vi "Multichannel Recording0.9EP.vi"() -> ()   [LabVIEW 2014]
uses:
  Consumer Data_ Consumer Event Com.ctl
  Data Producer States.ctl
  Enum State Typedef.ctl
  <vilib>/_DAQmxBase/Internals/DAQmxBase Read (Analog 2D DBL NChan NSamp).vi
  <vilib>/_DAQmxBase/Internals/DAQmxBase Create Channel (AI-Voltage-Basic).vi
  <vilib>/_DAQmxBase/Internals/DAQmxBase Timing (Sample Clock).vi
panel:
  out "Recording Progress (% )":dbl(slide) scale=0.0..1.0
  in  "Display Size":T1(ring)
  out "Data Producer State":T2=enum."Default"
  out "Data Consumer State":T3=enum."Default"
  in  "Open Button":bool
  in  "Tab Control":T4(tab)
  in  "Amplifier Channel 0":T5 {"Amplifier Model" items=["Select a Model", "AM 1700", "BMA 200"]}
  out "Channel 0 Graph":waveform(dbl)(graph)
  in  "User Data Channel 0":T6
  in  "Use Channel 0":bool caption="In Use?"
  out "Channel 1 Graph":waveform(dbl)(graph)
  in  "User Data Channel 1":T6
  in  "Amplifier Channel 1":T5 {"Amplifier Model" items=["Select a Model", "AM 1700", "BMA 200"]}
  in  "Use Channel 1":bool caption="In Use?"
  out "Channel 2 Graph":waveform(dbl)(graph)
  in  "User Data Channel 2":T6
  in  "Amplifier Channel 2":T5 {"Amplifier Model" items=["Select a Model", "AM 1700", "BMA 200"]}
  in  "Use Channel 2":bool caption="In Use?"
  out "Channel 3 Graph":waveform(dbl)(graph)
  in  "User Data Channel 3":T6
  in  "Amplifier Channel 3":T5 {"Amplifier Model" items=["Select a Model", "AM 1700", "BMA 200"]}
  in  "Use Channel 3":bool caption="In Use?"
  out "Overview Graph":waveform(dbl)[](graph)
  in  "Stop Preview":bool
  in  "OK Button":bool
  in  "Clear Display":bool
  in  "Preview Button":bool
  in  "Recording Time (s)":dbl
  in  "Sample Rate":i64=1000
  in  "Stop Button":bool
  out "Start Time hr/min":string
  out "Date mm/dd/yy":string
  in  "Exit Button":bool
  in  "Record Button":bool
  # "MSU EFISH Lab Multi-Channel Electronic Pulse Recorder v0.9E (Beta 6)"
  # "Setup"
  # "Must set sample rate before you press start"
  # "Preview"
  # "Recording"
  # "Blue for On\nOrange for Off"
  # "DC"
  # "AC"
  # "Blue for AC and Orange for DC"
  # "Blue for On\nOrange for Off"
  # "DC"
  # "AC"
  # "Blue for AC and Orange for DC"
  # "Blue for On\nOrange for Off"
  # "DC"
  # "AC"
  # "Blue for AC and Orange for DC"
  # "Blue for On\nOrange for Off"
  # "DC"
  # "AC"
  # "Blue for AC and Orange for DC"
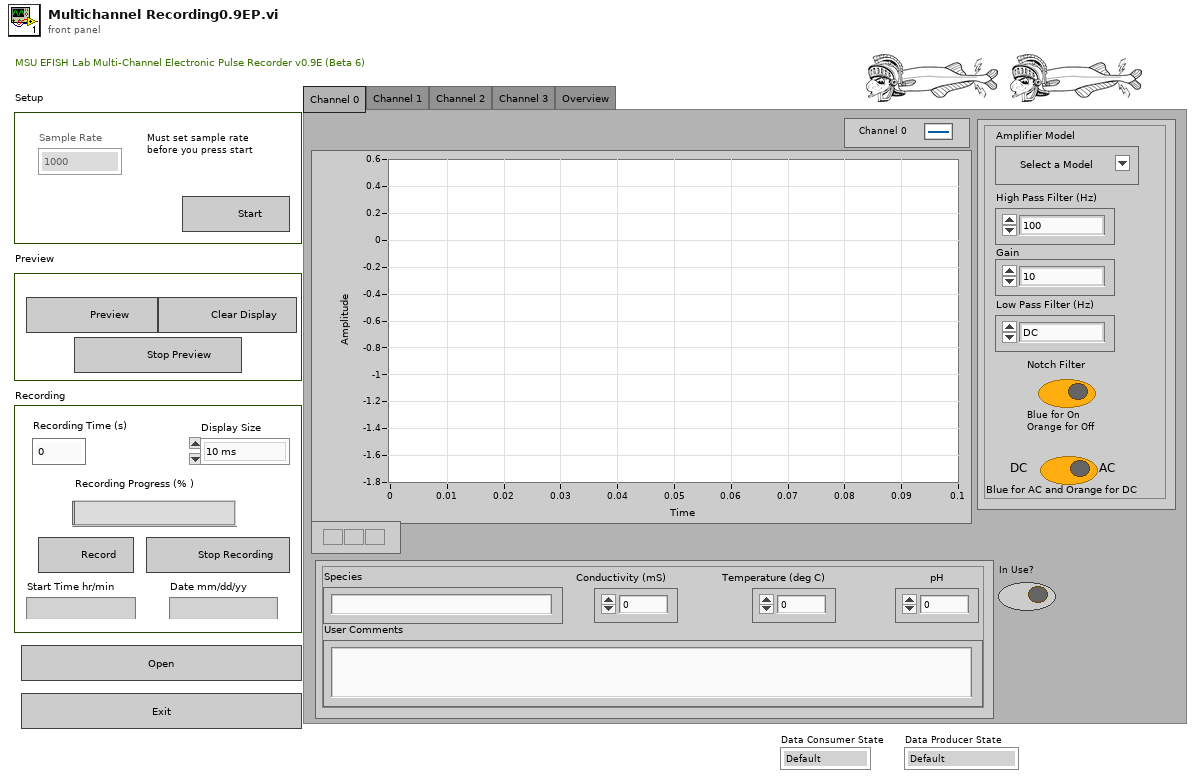
[diagram p1: front panel]
types:
  T1 = enum16{"10 ms", "100 ms", "1 Second", "10 sec", "30 sec"}
  T2 = typedef "Data Producer States.ctl" = enum16{"Read Data", "Set Sample Clock", "Default", "Exit", "Preview"}
  T3 = typedef "Consumer Data_ Consumer Event Com.ctl" = enum16{"Recording", "Create File", "Clear Memory", "Default", "End File", "Exit", "Set Sample Clock", "Preview"}
  T4 = enum32{"Channel 0", "Channel 1", "Channel 2", "Channel 3", "Overview"}
  T5 = cluster{"Low Pass Filter (Hz)":enum16{"DC", "0.1", "1", "3", "10", "30", "100", "300"}, "Gain ":enum16{"10", "20", "50", "100", "200", "500", "1000", "2k", "5k", "10k", "20k", "50k"}, "High Pass Filter (Hz)":enum16{"100", "500", "1000", "3000", "5000", "10,000", "20,000", "30,000", "50,000"}, "Notch Filter":bool, "Amplifier Model":u16, "AC/DC Switch":bool}
  T6 = cluster{"pH":dbl, "Conductivity (mS)":dbl, "Temperature (deg C)":dbl, "User Comments":string, "Species":string}
  T7 = enum8{"Enabled", "Disabled", "Disabled and Grayed Out"}
  T8 = cluster{"Overview Graph":refnum<vi>, "Channel 3 Graph":refnum<vi>, "Channel 2 Graph":refnum<vi>, "Channel 1 Graph":refnum<vi>, "Channel 0 Graph":refnum<vi>}
  T9 = typedef "Enum State Typedef.ctl" = enum16{"Default", "Open FIle", "Beginning State", "Set the Sample Clock", "Prepreview Handling", "Clear Display", "Preview Data", "Stop", "Exit", "Record", "Create File"}
  T10 = enum16{"Recording", "Create File", "Clear Memory", "Default"}
  T11 = cluster{"Refnum out":refnum<k34>, "Refnum out":refnum<k34>, "Refnum out":refnum<k34>, "Refnum out":refnum<k34>}
  T12 = cluster{"Use Channel 0":bool, "Use Channel 1":bool, "Use Channel 2":bool, "Use Channel 3":bool}
  T13 = cluster{"Waveform":waveform(dbl), "Waveform":waveform(dbl), "Waveform":waveform(dbl), "Waveform":waveform(dbl), waveform(dbl)[]}
  T14 = cluster{"tdms file out":refnum<k34>, "tdms file out":refnum<k34>, "tdms file out":refnum<k34>, "tdms file out":refnum<k34>}
  T15 = cluster{"User Data Channel 0":cluster{"pH":dbl, "Conductivity (mS)":dbl, "Temperature (deg C)":dbl, "User Comments":string, "Species":string}, "Amplifier Channel 0":cluster{"Low Pass Filter (Hz)":enum16{"DC", "0.1", "1", "3", "10", "30", "100", "300"}, "Gain ":enum16{"10", "20", "50", "100", "200", "500", "1000", "2k", "5k", "10k", "20k", "50k"}, "High Pass Filter (Hz)":enum16{"100", "500", "1000", "3000", "5000", "10,000", "20,000", "30,000", "50,000"}, "Notch Filter":bool, "Amplifier Model":u16, "AC/DC Switch":bool}, "User Data Channel 1":cluster{"pH":dbl, "Conductivity (mS)":dbl, "Temperature (deg C)":dbl, "User Comments":string, "Species":string}, "Amplifier Channel 1":cluster{"Low Pass Filter (Hz)":enum16{"DC", "0.1", "1", "3", "10", "30", "100", "300"}, "Gain ":enum16{"10", "20", "50", "100", "200", "500", "1000", "2k", "5k", "10k", "20k", "50k"}, "High Pass Filter (Hz)":enum16{"100", "500", "1000", "3000", "5000", "10,000", "20,000", "30,000", "50,000"}, "Notch Filter":bool, "Amplifier Model":u16, "AC/DC Switch":bool}, "User Data Channel 2":cluster{"pH":dbl, "Conductivity (mS)":dbl, "Temperature (deg C)":dbl, "User Comments":string, "Species":string}, "Amplifier Channel 2":cluster{"Low Pass Filter (Hz)":enum16{"DC", "0.1", "1", "3", "10", "30", "100", "300"}, "Gain ":enum16{"10", "20", "50", "100", "200", "500", "1000", "2k", "5k", "10k", "20k", "50k"}, "High Pass Filter (Hz)":enum16{"100", "500", "1000", "3000", "5000", "10,000", "20,000", "30,000", "50,000"}, "Notch Filter":bool, "Amplifier Model":u16, "AC/DC Switch":bool}, "User Data Channel 3":cluster{"pH":dbl, "Conductivity (mS)":dbl, "Temperature (deg C)":dbl, "User Comments":string, "Species":string}, "Amplifier Channel 3":cluster{"Low Pass Filter (Hz)":enum16{"DC", "0.1", "1", "3", "10", "30", "100", "300"}, "Gain ":enum16{"10", "20", "50", "100", "200", "500", "1000", "2k", "5k", "10k", "20k", "50k"}, "High Pass Filter (Hz)":enum16{"100", "500", "1000", "3000", "5000", "10,000", "20,000", "30,000", "50,000"}, "Notch Filter":bool, "Amplifier Model":u16, "AC/DC Switch":bool}}
  T16 = enum16{"Read Data", "Set Sample Clock", "Default", "Exit"}
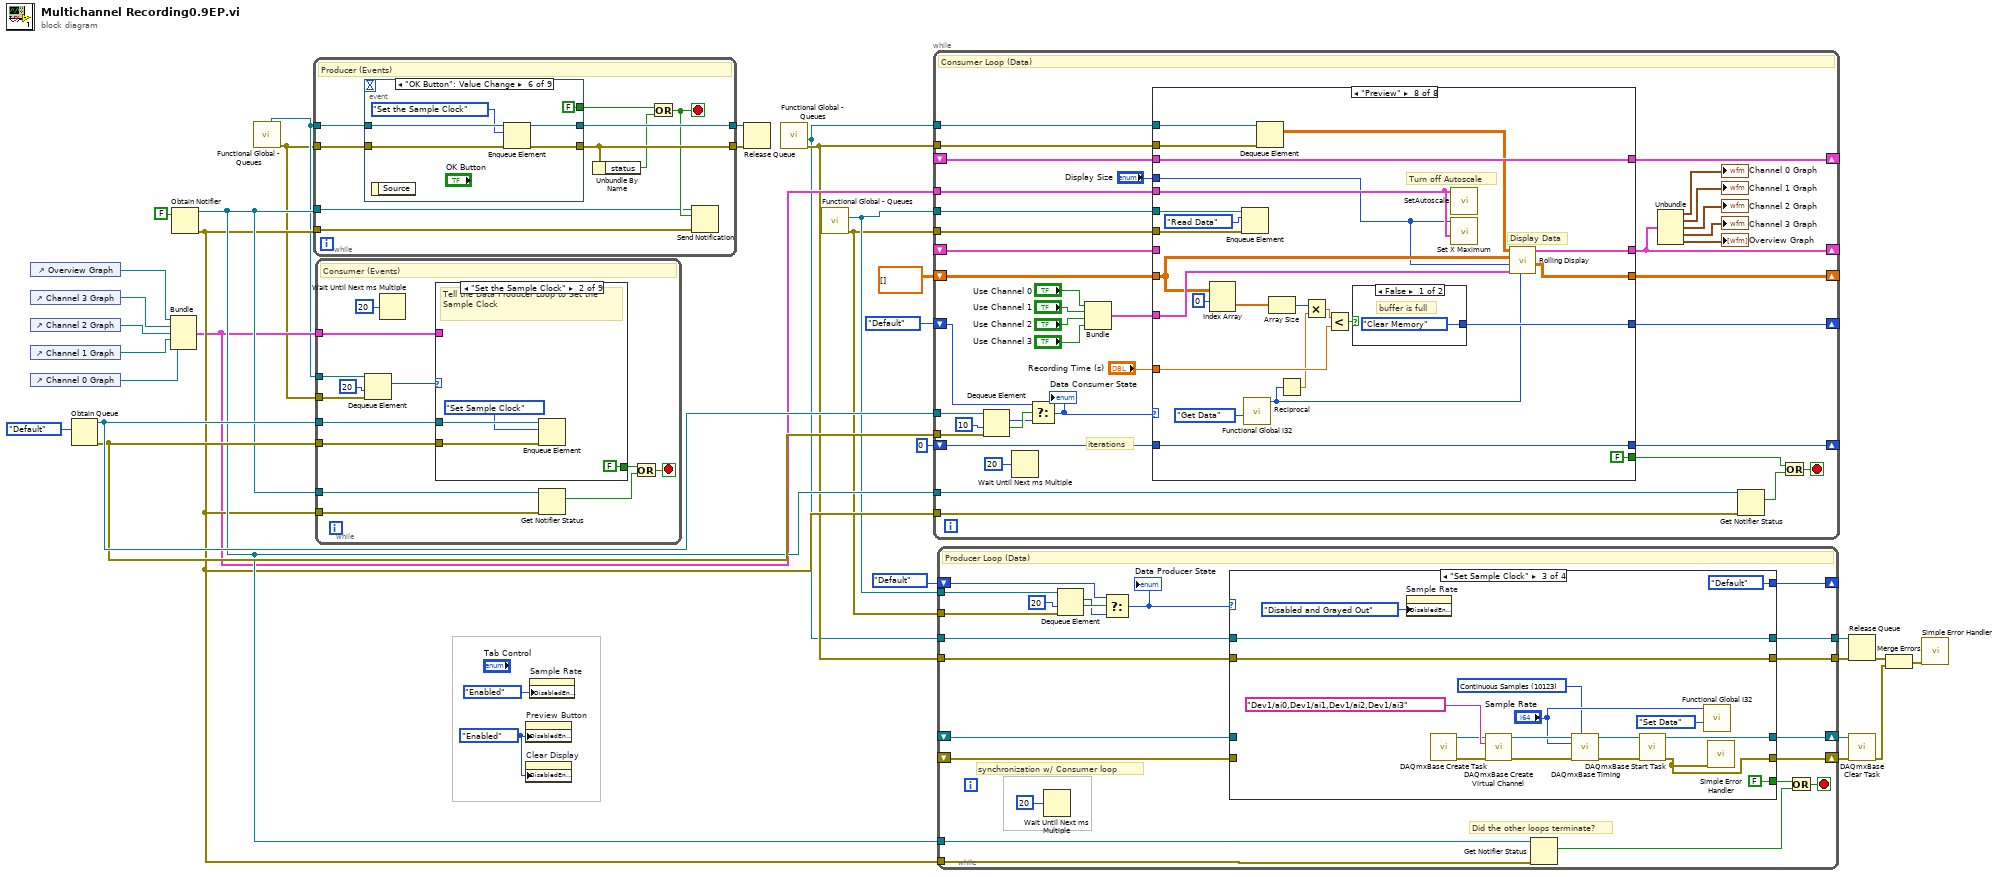
[diagram p0: block diagram]
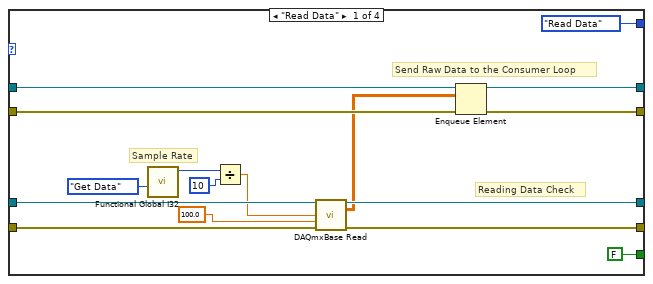
[diagram p2: hidden frame]
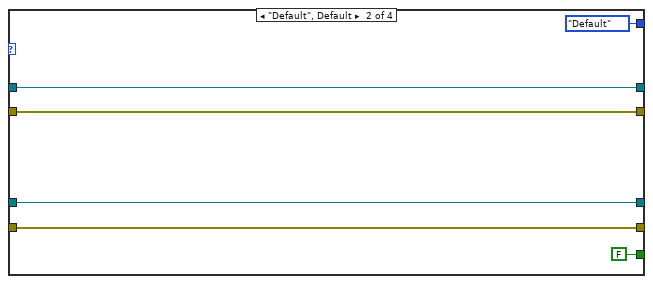
[diagram p3: hidden frame]
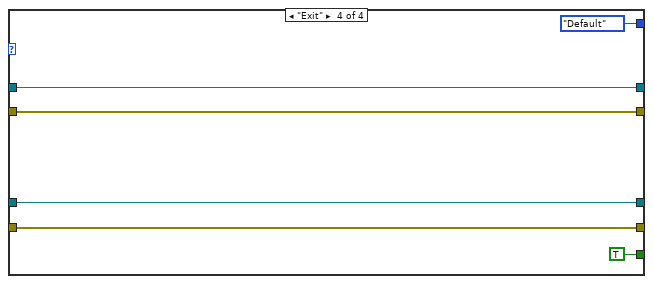
[diagram p4: hidden frame]
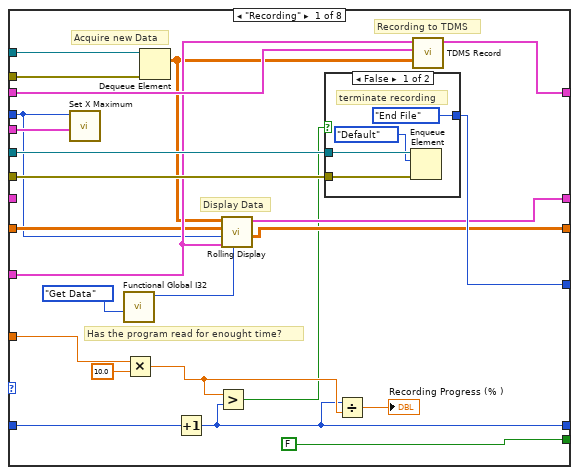
[diagram p5: hidden frame]
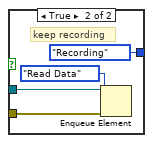
[diagram p6: hidden frame]
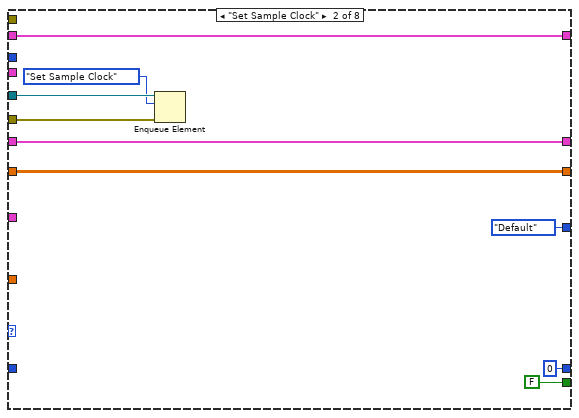
[diagram p7: hidden frame]
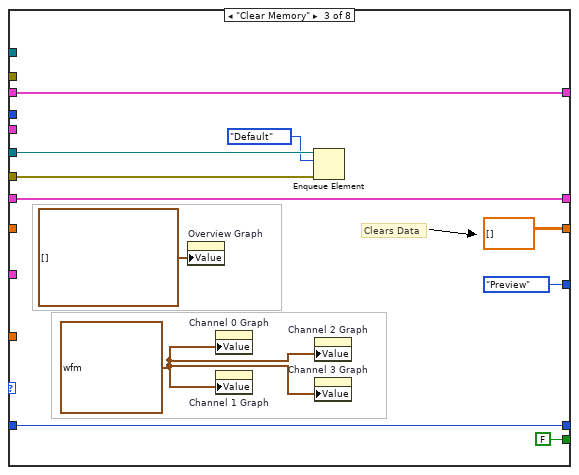
[diagram p8: hidden frame]
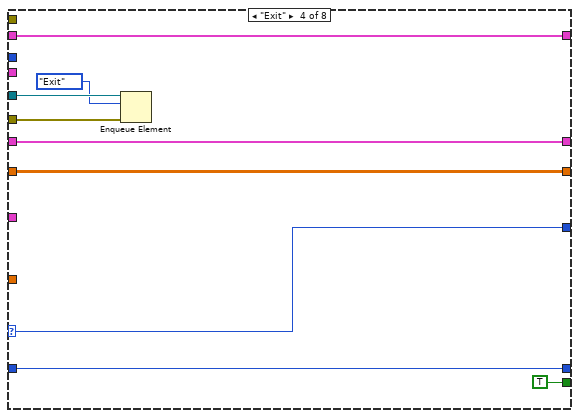
[diagram p9: hidden frame]
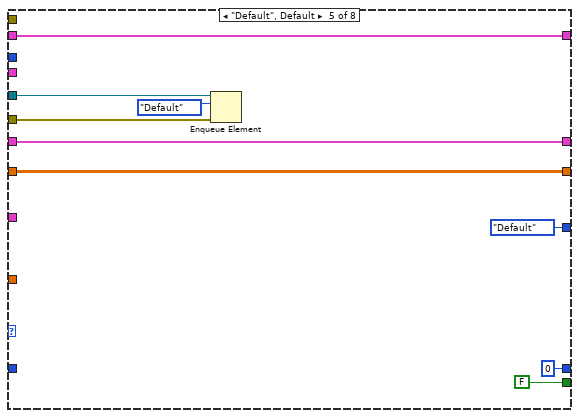
[diagram p10: hidden frame]
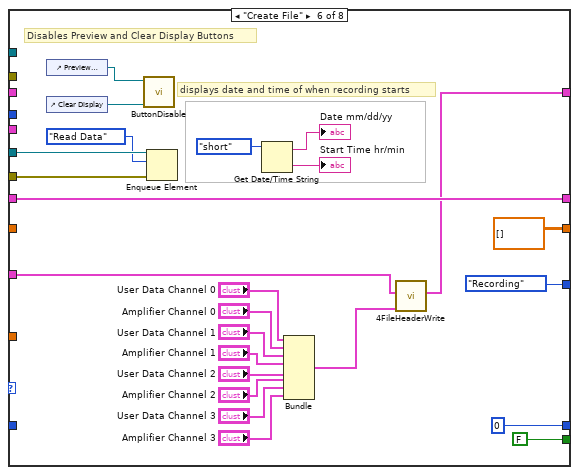
[diagram p11: hidden frame]
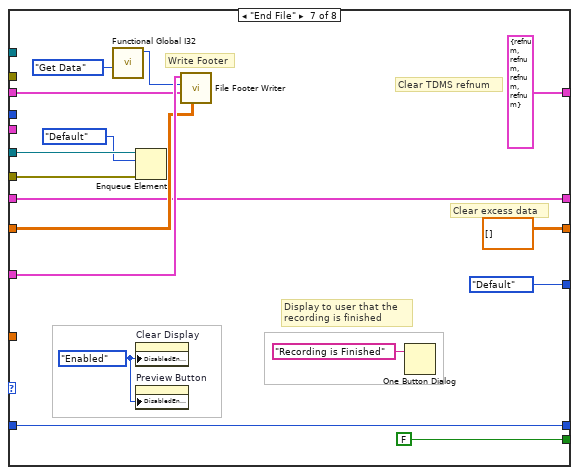
[diagram p12: hidden frame]
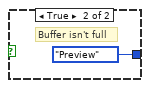
[diagram p13: hidden frame]
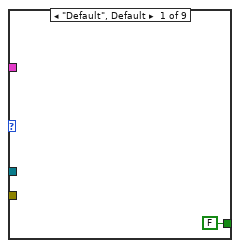
[diagram p14: hidden frame]
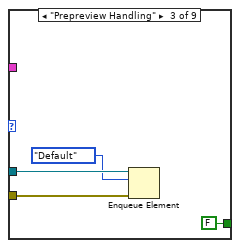
[diagram p15: hidden frame]
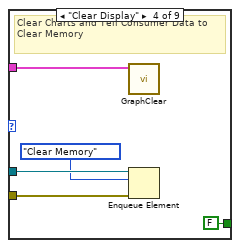
[diagram p16: hidden frame]
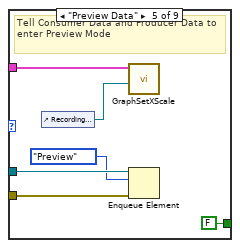
[diagram p17: hidden frame]
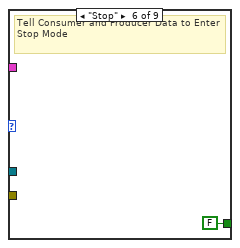
[diagram p18: hidden frame]
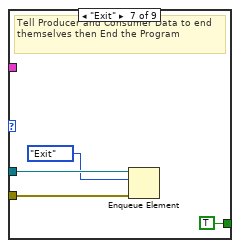
[diagram p19: hidden frame]
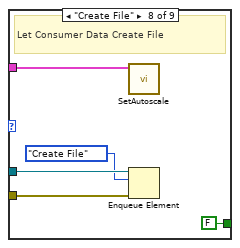
[diagram p20: hidden frame]
diagram:
  w13 = T7."Enabled" ("Disabled")
  n1 = control-ref of="Overview Graph"() -> (w12:refnum<vi>)
  n2 = control-ref of="Channel 3 Graph"() -> (w11:refnum<vi>)
  n3 = control-ref of="Channel 2 Graph"() -> (w10:refnum<vi>)
  n4 = control-ref of="Channel 1 Graph"() -> (w9:refnum<vi>)
  n5 = control-ref of="Channel 0 Graph"() -> (w8:refnum<vi>)
  n6 = Obtain Queue(element data type=Consumer_Data__Consumer_Event_Com."Default") -> (queue out=w29:refnum<queue>, error out=w28:errorcluster)  [unwired: 4 in, 1 out]
  n7 = Bundle("Overview Graph"=w12, "Channel 3 Graph"=w11, "Channel 2 Graph"=w10, "Channel 1 Graph"=w9, "Channel 0 Graph"=w8) -> (w7:T8)  [unwired: 1 in]
  n8 = Obtain Notifier(notification data type=FALSE) -> (notifier out=w15:refnum<notifier>, error out=w14:errorcluster)  [unwired: 3 in, 1 out]
  n9 = call "Functional Global - Queues.vi"() -> ("Error Out"=w1:errorcluster, "Producer Consumer Events Q"=w2:refnum<queue>)  [unwired: 7 in, 3 out]
  n10 = while {
    tunnel: w2 -> [w42]
    tunnel: w1 -> [w41]
    tunnel: [w40] -> w33
    tunnel: [w39] -> w32
    tunnel: w15 -> [w35]
    tunnel: w14 -> [w34]
    stop <- w36 stop-if-true
    # "Producer (Events)"
    n11 = event shown="[5] \"OK Button\": Value Change" {
      selector: _ -> [_ _ _ _ _ _ _ _ _]
      dyn-events: _ -> [_ _ _ _ _ _ _ _ _]
      timeout: _ -> [_ _ _ _ _ _ _ _ _]
      tunnel: [FALSE ("Exit Button") "Exit Button" FALSE ("Exit Button") FALSE ("Exit Button") FALSE ("Exit Button") FALSE ("Exit Button") FALSE ("Exit Button") FALSE ("Exit Button") FALSE ("Exit Button")] -> w38
      tunnel: w42 -> [w44 w50 w57 w63 w69 w75 w81 w87 w93]
      tunnel: w41 -> [w43 w49 w56 w62 w68 w74 w80 w86 w92]
      tunnel: [w44 w47 w53 w59 w65 w71 w77 w83 w89] -> w40
      tunnel: [w43 w46 w52 w58 w64 w70 w76 w82 w88] -> w39
      event Timeout {
        n12 = event-data() -> ()  [unwired: 1 in, 1 out]
      }
      event "Exit Button": Value Change {
        n13 = event-data() -> ()  [unwired: 1 in, 1 out]
        n14 = Enqueue Element(queue=w50, element=Enum_State_Typedef."Exit", error in (no error)=w49) -> (queue out=w47:refnum<queue>, error out=w46:errorcluster)  [unwired: 1 in, 1 out]
      }
      event "Preview Button": Value Change {
        n15 = event-data() -> ()  [unwired: 1 in, 1 out]
        n16 = Enqueue Element(queue=w57, element=Enum_State_Typedef."Preview Data", error in (no error)=w56) -> (queue out=w53:refnum<queue>, error out=w52:errorcluster)  [unwired: 1 in, 1 out]
      }
      event "Stop Preview": Value Change {
        n17 = event-data() -> ()  [unwired: 1 in, 1 out]
        n18 = Enqueue Element(queue=w63, element=Enum_State_Typedef."Prepreview Handling", error in (no error)=w62) -> (queue out=w59:refnum<queue>, error out=w58:errorcluster)  [unwired: 1 in, 1 out]
      }
      event "Open Button": Value Change {
        n19 = event-data() -> ()  [unwired: 1 in, 1 out]
        n20 = Enqueue Element(queue=w69, element=Enum_State_Typedef."Open FIle", error in (no error)=w68) -> (queue out=w65:refnum<queue>, error out=w64:errorcluster)  [unwired: 1 in, 1 out]
      }
      event "OK Button": Value Change {
        n21 = event-data() -> ()  [unwired: 1 in, 1 out]
        n22 = Enqueue Element(queue=w75, element=Enum_State_Typedef."Set the Sample Clock", error in (no error)=w74) -> (queue out=w71:refnum<queue>, error out=w70:errorcluster)  [unwired: 1 in, 1 out]
      }
      event "Stop Button": Value Change {
        n23 = event-data() -> ()  [unwired: 1 in, 1 out]
        n24 = Enqueue Element(queue=w81, element=Enum_State_Typedef."Stop", error in (no error)=w80) -> (queue out=w77:refnum<queue>, error out=w76:errorcluster)  [unwired: 1 in, 1 out]
      }
      event "Record Button": Value Change {
        n25 = event-data() -> ()  [unwired: 1 in, 1 out]
        n26 = Enqueue Element(queue=w87, element=Enum_State_Typedef."Create File", error in (no error)=w86) -> (queue out=w83:refnum<queue>, error out=w82:errorcluster)  [unwired: 1 in, 1 out]
      }
      event "Clear Display": Value Change {
        n27 = event-data() -> ()  [unwired: 1 in, 1 out]
        n28 = Enqueue Element(queue=w93, element=Enum_State_Typedef."Clear Display", error in (no error)=w92) -> (queue out=w89:refnum<queue>, error out=w88:errorcluster)  [unwired: 1 in, 1 out]
      }
    }
    n29 = Unbundle By Name(w39) -> ("status"=w37:bool)
    n30 = Or(x=w38, y=w37) -> (x .or. y?=w36:bool)
    n31 = Send Notification(notification=w36, notifier=w35, error in (no error)=w34) -> ()  [unwired: 2 out]
  }
  n32 = while {
    tunnel: w2 -> [w106]
    tunnel: w1 -> [w105]
    tunnel: w29 -> [w104]
    tunnel: w28 -> [w103]
    tunnel: w15 -> [w98]
    tunnel: w14 -> [w97]
    tunnel: w7 -> [w94]
    stop <- w96 stop-if-true
    # "Consumer (Events)"
    n33 = Dequeue Element(queue=w106, timeout in ms (-1)=20, error in (no error)=w105) -> (element=w101:T9)  [unwired: 3 out]
    n34 = Wait Until Next ms Multiple(millisecond multiple=u32 20) -> ()  [unwired: 1 out]
    n35 = case shown="\"Set the Sample Clock\"" w101 {
      tunnel: w104 -> [_ w110 w114 w119 w125 _ w131 w135 _]
      tunnel: w103 -> [_ w109 w113 w118 w124 _ w130 w134 _]
      tunnel: [FALSE FALSE FALSE FALSE FALSE FALSE TRUE FALSE FALSE] -> w102
      tunnel: w94 -> [_ _ _ w116 w121 _ _ w132 _]
      frame "Default", Default {
      }
      frame "Set the Sample Clock" {
        # "Tell the Data Producer Loop to Set the Sample Clock"
        n36 = Enqueue Element(queue=w110, element=Consumer_Data__Consumer_Event_Com."Set Sample Clock", error in (no error)=w109) -> ()  [unwired: 1 in, 3 out]
      }
      frame "Prepreview Handling" {
        n37 = Enqueue Element(queue=w114, element=Consumer_Data__Consumer_Event_Com."Default", error in (no error)=w113) -> ()  [unwired: 1 in, 3 out]
      }
      frame "Clear Display" {
        # "Clear Charts and Tell Consumer Data to Clear Memory"
        n38 = call "GraphClear.vi"("Graph Reference Cluster"=w116) -> ()  [unwired: 11 in]
        n39 = Enqueue Element(queue=w119, element=Consumer_Data__Consumer_Event_Com."Clear Memory", error in (no error)=w118) -> ()  [unwired: 1 in, 3 out]
      }
      frame "Preview Data" {
        # "Tell Consumer Data and Producer Data to enter Preview Mode"
        n40 = control-ref of="Recording Time (s)"() -> (w122:refnum<vi>)
        n41 = call "GraphSetXScale.vi"("Graph Reference Cluster"=w121, "Recording Time Reference"=w122) -> ()  [unwired: 9 in]
        n42 = Enqueue Element(queue=w125, element=Consumer_Data__Consumer_Event_Com."Preview", error in (no error)=w124) -> ()  [unwired: 1 in, 3 out]
      }
      frame "Stop" {
        # "Tell Consumer and Producer Data to Enter Stop Mode"
      }
      frame "Exit" {
        # "Tell Producer and Consumer Data to end themselves then End the Program"
        n43 = Enqueue Element(queue=w131, element=Consumer_Data__Consumer_Event_Com."Exit", error in (no error)=w130) -> ()  [unwired: 1 in, 3 out]
      }
      frame "Create File" {
        # "Let Consumer Data Create File"
        n44 = call "SetAutoscale.vi"("Graph Reference Cluster"=w132) -> ()  [unwired: 11 in]
        n45 = Enqueue Element(queue=w135, element=Consumer_Data__Consumer_Event_Com."Create File", error in (no error)=w134) -> ()  [unwired: 1 in, 3 out]
      }
      frame "Open FIle" {
        # "Tell the Data Consumer to Create the File"
        n46 = call "File Dialog"() -> ("selected path"=w137:path)  [unwired: 12 in, 3 out]
        n47 = call <vilib>:"TDMS - File Viewer.vi"("file path"=w137) -> ()  [unwired: 5 in, 2 out]
      }
    }
    n48 = Get Notifier Status(notifier=w98, error in (no error)=w97) -> (current notification=w95:bool)  [unwired: 4 out]
    n49 = Or(x=w102, y=w95) -> (x .or. y?=w96:bool)
  }
  n50 = property on="Preview Button" class="Bool (strict)"("DisabledEnum"=w13) -> ()  [unwired: 2 in, 2 out]
  n51 = property on="Clear Display" class="Bool"("DisabledEnum"=w13) -> ()  [unwired: 2 in, 2 out]
  n52 = property on="Sample Rate" class="DigNum (strict)"("DisabledEnum"=T7."Enabled" ("Disabled")) -> ()  [unwired: 2 in, 2 out]
  n53 = Release Queue(queue=w33, error in (no error)=w32) -> ()  [unwired: 1 in, 3 out]
  n54 = call "Functional Global - Queues.vi"() -> ("Error Out"=w6:errorcluster, "Data Q"=w5:refnum<queue>)  [unwired: 7 in, 3 out]
  n55 = call "Functional Global - Queues.vi"() -> ("Error Out"=w3:errorcluster, "Data Producer Control Q"=w4:refnum<queue>)  [unwired: 7 in, 3 out]
  n56 = while {
    tunnel: w5 -> [w170]
    tunnel: w6 -> [w169]
    tunnel: w29 -> [w177]
    tunnel: w28 -> [w176]
    shift-right: [w171] -> _
    shift-left: Consumer_Data__Consumer_Event_Com."Default" -> [w172]
    shift-right: [w165] -> _
    shift-left: dbl[][] [] -> [w168]
    shift-right: [w164] -> _
    shift-left: _ -> [w163]
    tunnel: w4 -> [w161]
    tunnel: w3 -> [w160]
    shift-right: [w156] -> _
    shift-left: 0 -> [w158]
    tunnel: w15 -> [w150]
    tunnel: w14 -> [w149]
    shift-right: [w142] -> _
    shift-left: _ -> [w141]
    tunnel: w7 -> [w139]
    stop <- w152 stop-if-true
    # "iterations"
    # "Consumer Loop (Data)"
    n57 = Dequeue Element(queue=w177, timeout in ms (-1)=10, error in (no error)=w176) -> (element=w174:T3, timed out?=w175:bool)  [unwired: 2 out]
    n58 = Wait Until Next ms Multiple(millisecond multiple=u32 20) -> ()  [unwired: 1 out]
    n59 = Select(t=w172, s=w175, f=w174) -> (s? t:f=w173:T3)
    "Data Consumer State" <- w173
    n60 = Bundle("Use Channel 0"="Use Channel 0", "Use Channel 1"="Use Channel 1", "Use Channel 2"="Use Channel 2", "Use Channel 3"="Use Channel 3") -> (w166:T12)  [unwired: 1 in]
    n61 = case shown="\"Preview\"" w173 {
      selector: w173 -> [_ _ _ w236 _ _ _ _]
      tunnel: [w194 Consumer_Data__Consumer_Event_Com."Default" Consumer_Data__Consumer_Event_Com."Preview" w236 T10."Default" Consumer_Data__Consumer_Event_Com."Recording" Consumer_Data__Consumer_Event_Com."Default" w306] -> w171
      tunnel: w170 -> [w200 _ _ _ _ _ _ w312]
      tunnel: w169 -> [w199 _ _ _ _ _ _ w311]
      tunnel: [FALSE FALSE FALSE TRUE FALSE FALSE FALSE FALSE] -> w151
      tunnel: w168 -> [w180 w215 _ w237 w245 _ w285 w293]
      tunnel: w166 -> [w189 _ _ _ _ w250 w287 w298]
      tunnel: [w187 w215 dbl[][] [] ("Output Decimated Data") w237 w245 dbl[][] [] ("Output Decimated Data") dbl[][] [] ("Output Data") w296] -> w165
      tunnel: [w198 w214 w226 w235 w244 w252 T11 {"Refnum out"=refnum, "Refnum out"=refnum, "Refnum out"=refnum, "Refnum out"=refnum} ("Output TDMS File Cluster") w299] -> w164
      tunnel: w163 -> [w191 w214 w226 w235 w244 _ w286 w299]
      tunnel: w161 -> [w193 w218 w225 w234 w242 w265 w280 w304]
      tunnel: w160 -> [w192 w217 w224 w233 w241 w264 w279 w303]
      tunnel: w158 -> [w197 _ w222 w231 _ _ w277 w301]
      tunnel: "Recording Time (s)" -> [w196 _ _ _ _ _ _ w294]
      tunnel: [w183 0 w222 w231 0 0 w277 w301] -> w156
      tunnel: [w188 w210 w221 w230 w239 w261 w275 w297] -> w142
      tunnel: w141 -> [_ w210 w221 w230 w239 w261 w275 _]
      tunnel: "Display Size" -> [w179 _ _ _ _ _ _ w290]
      tunnel: w139 -> [w185 _ _ _ _ _ _ w295]
      frame "Recording" {
        # "Acquire new Data"
        # "Has the program read for enought time?"
        # "Display Data"
        # "Recording to TDMS"
        n62 = call "Set X Maximum.vi"("Graph Reference Cluster"=w185, "Display Size"=w179) -> ()  [unwired: 10 in]
        n63 = call "Functional Global I32.vi"("Enum"=enum16{"Set Data", "Get Data"}."Get Data") -> ("Integer"=w178:i32)  [unwired: 10 in]
        n64 = Multiply(x=w196, y=10.0) -> (x*y=w184:dbl)
        n65 = Dequeue Element(queue=w200, error in (no error)=w199) -> (element=w181:dbl[][])  [unwired: 1 in, 3 out]
        n66 = Increment(x=w197) -> (x+1=w183:i32)
        n67 = Greater?(x=w184, y=w183) -> (0:w182:bool)
        n68 = call "Rolling Display.vi"("Sample Rate"=w178, "Channels in Use"=w189, "Display Size"=w179, "Old Data"=w180, "Input Data"=w181) -> ("Output Array Values"=w187:dbl[][], "Output Waveform Cluster"=w188:T13)  [unwired: 5 in]
        n69 = case shown="False" w182 {
          tunnel: [Consumer_Data__Consumer_Event_Com."End File" Consumer_Data__Consumer_Event_Com."Recording"] -> w194
          tunnel: w193 -> [w204 w208]
          tunnel: w192 -> [w203 w207]
          frame False {
            # "terminate recording"
            n70 = Enqueue Element(queue=w204, element=Data_Producer_States."Default", error in (no error)=w203) -> ()  [unwired: 1 in, 3 out]
          }
          frame True {
            # "keep recording"
            n71 = Enqueue Element(queue=w208, element=Data_Producer_States."Read Data", error in (no error)=w207) -> ()  [unwired: 1 in, 3 out]
          }
        }
        n72 = Divide(x=w183, y=w184) -> (x/y=→"Recording Progress (% )":dbl)
        n73 = call "TDMS Record.vi"("Data"=w181, "Input TDMS File Cluster"=w191, "In Use Cluster"=w189) -> ("Output TDMS File Cluster"=w198:T14)  [unwired: 8 in]
      }
      frame "Set Sample Clock" {
        n74 = Enqueue Element(queue=w218, element=Data_Producer_States."Set Sample Clock", error in (no error)=w217) -> ()  [unwired: 1 in, 3 out]
      }
      frame "Clear Memory" {
        w220 = waveform(dbl) {"t0"=timestamp(0 s since 1904-01-01), "dt"=1.0, "Y"=[]} ("Channel 0 Graph")
        # "Clears Data"
        n75 = property on="Overview Graph" class="WFGraph (strict)"("Value"=waveform(dbl)[] [] ("Overview Graph")) -> ()  [unwired: 2 in, 2 out]
        n76 = property on="Channel 0 Graph" class="WFGraph (strict)"("Value"=w220) -> ()  [unwired: 2 in, 2 out]
        n77 = property on="Channel 1 Graph" class="WFGraph (strict)"("Value"=w220) -> ()  [unwired: 2 in, 2 out]
        n78 = Enqueue Element(queue=w225, element=Data_Producer_States."Default", error in (no error)=w224) -> ()  [unwired: 1 in, 3 out]
        n79 = property on="Channel 2 Graph" class="WFGraph (strict)"("Value"=w220) -> ()  [unwired: 2 in, 2 out]
        n80 = property on="Channel 3 Graph" class="WFGraph (strict)"("Value"=w220) -> ()  [unwired: 2 in, 2 out]
      }
      frame "Exit" {
        n81 = Enqueue Element(queue=w234, element=Data_Producer_States."Exit", error in (no error)=w233) -> ()  [unwired: 1 in, 3 out]
      }
      frame "Default", Default {
        n82 = Enqueue Element(queue=w242, element=Data_Producer_States."Default", error in (no error)=w241) -> ()  [unwired: 1 in, 3 out]
      }
      frame "Create File" {
        # "displays date and time of when recording starts"
        # "Disables Preview and Clear Display Buttons"
        n83 = control-ref of="Preview Button"() -> (w248:refnum<vi>)
        n84 = control-ref of="Clear Display"() -> (w249:refnum<vi>)
        n85 = call "ButtonDisable.vi"("Clear Display Button Reference"=w249, "Preview Button Reference"=w248) -> ()  [unwired: 10 in]
        n86 = Enqueue Element(queue=w265, element=Data_Producer_States."Read Data", error in (no error)=w264) -> ()  [unwired: 1 in, 3 out]
        n87 = Get Date/Time String(date format (0)=enum16{"short", "long", "abbreviated"}."short") -> (date string=→"Date mm/dd/yy":string, time string=→"Start Time hr/min":string)  [unwired: 2 in]
        n88 = Bundle("User Data Channel 0"="User Data Channel 0", "Amplifier Channel 0"="Amplifier Channel 0", "User Data Channel 1"="User Data Channel 1", "Amplifier Channel 1"="Amplifier Channel 1", "User Data Channel 2"="User Data Channel 2", "Amplifier Channel 2"="Amplifier Channel 2", "User Data Channel 3"="User Data Channel 3", "Amplifier Channel 3"="Amplifier Channel 3") -> (w251:T15)  [unwired: 1 in]
        n89 = call "4FileHeaderWrite.vi"("MetaData Cluster"=w251, "In Use Cluster"=w250) -> ("Cluster out"=w252:T11)  [unwired: 9 in]
      }
      frame "End File" {
        w274 = T7."Enabled" ("Disabled")
        # "Write Footer"
        # "Clear TDMS refnum"
        # "Clear excess data"
        # "Display to user that the \nrecording is finished"
        n90 = call "Functional Global I32.vi"("Enum"=enum16{"Set Data", "Get Data"}."Get Data") -> ("Integer"=w272:i32)  [unwired: 10 in]
        n91 = Enqueue Element(queue=w280, element=Data_Producer_States."Default", error in (no error)=w279) -> ()  [unwired: 1 in, 3 out]
        n92 = property on="Clear Display" class="Bool"("DisabledEnum"=w274) -> ()  [unwired: 2 in, 2 out]
        n93 = property on="Preview Button" class="Bool (strict)"("DisabledEnum"=w274) -> ()  [unwired: 2 in, 2 out]
        n94 = call "File Footer Writer.vi"("Old Data"=w285, "TDMS File Cluster"=w286, "Sample Rate"=w272, "In Use Cluster"=w287) -> ()  [unwired: 8 in]
        n95 = One Button Dialog(message="Recording is Finished") -> ()  [unwired: 1 in, 1 out]
      }
      frame "Preview" {
        # "Display Data"
        # "Turn off Autoscale"
        n96 = Index Array(array=w293, index (row)=0) -> (element=w309:dbl[])  [unwired: 1 in]
        n97 = Enqueue Element(queue=w304, element=Data_Producer_States."Read Data", error in (no error)=w303) -> ()  [unwired: 1 in, 3 out]
        n98 = call "Functional Global I32.vi"("Enum"=enum16{"Set Data", "Get Data"}."Get Data") -> ("Integer"=w291:i32)  [unwired: 10 in]
        n99 = Dequeue Element(queue=w312, error in (no error)=w311) -> (element=w292:dbl[][])  [unwired: 1 in, 3 out]
        n100 = Array Size(array=w309) -> (size(s)=w288:i32)
        n101 = Reciprocal(x=w291) -> (1/x=w289:dbl)
        n102 = Multiply(x=w288, y=w289) -> (x*y=w308:dbl)
        n103 = Less?(x=w308, y=w294) -> (x < y?=w307:bool)
        n104 = case shown="False" w307 {
          tunnel: [Consumer_Data__Consumer_Event_Com."Clear Memory" Consumer_Data__Consumer_Event_Com."Preview"] -> w306
          frame False {
            # "buffer is full"
          }
          frame True {
            # "Buffer isn't full"
          }
        }
        n105 = call "SetAutoscale.vi"("Graph Reference Cluster"=w295) -> ()  [unwired: 11 in]
        n106 = call "Set X Maximum.vi"("Graph Reference Cluster"=w295, "Display Size"=w290) -> ()  [unwired: 10 in]
        n107 = call "Rolling Display.vi"("Sample Rate"=w291, "Channels in Use"=w298, "Display Size"=w290, "Old Data"=w293, "Input Data"=w292) -> ("Output Array Values"=w296:dbl[][], "Output Waveform Cluster"=w297:T13)  [unwired: 5 in]
      }
    }
    n108 = Unbundle(w142) -> ("Waveform"=→"Channel 0 Graph":waveform(dbl), "Waveform"=→"Channel 1 Graph":waveform(dbl), "Waveform"=→"Channel 2 Graph":waveform(dbl), "Waveform"=→"Channel 3 Graph":waveform(dbl), →"Overview Graph":waveform(dbl)[])
    n109 = Get Notifier Status(notifier=w150, error in (no error)=w149) -> (current notification=w148:bool)  [unwired: 4 out]
    n110 = Or(x=w151, y=w148) -> (x .or. y?=w152:bool)
  }
  n111 = while {
    tunnel: w5 -> [w336]
    tunnel: w6 -> [w333]
    tunnel: [w335] -> w31
    tunnel: [w334] -> w30
    shift-right: [w321] -> _
    shift-left: Data_Producer_States."Default" -> [w316]
    shift-right: [w332] -> w26
    shift-left: _ -> [w330]
    shift-right: [w331] -> w25
    shift-left: _ -> [w329]
    tunnel: w4 -> [w326]
    tunnel: w3 -> [w325]
    tunnel: w15 -> [w318]
    tunnel: w14 -> [w317]
    stop <- w320 stop-if-true
    # "synchronization w/ Consumer loop"
    # "Did the other loops terminate?"
    # "Producer Loop (Data)"
    n112 = Wait Until Next ms Multiple(millisecond multiple=u32 20) -> ()  [unwired: 1 out]
    n113 = Dequeue Element(queue=w326, timeout in ms (-1)=20, error in (no error)=w325) -> (element=w315:T2, timed out?=w324:bool)  [unwired: 2 out]
    n114 = Select(t=w316, s=w324, f=w315) -> (s? t:f=w323:T2)
    "Data Producer State" <- w323
    n115 = case shown="\"Set Sample Clock\"" w323 {
      tunnel: w336 -> [w348 w358 w367 w377]
      tunnel: [w346 w358 w367 w377] -> w335
      tunnel: [w345 w357 w366 w378] -> w334
      tunnel: w333 -> [w347 w357 w366 w378]
      tunnel: [w350 w356 w368 w379] -> w332
      tunnel: [w349 w355 w359 w380] -> w331
      tunnel: w330 -> [w352 w356 _ w379]
      tunnel: w329 -> [w351 w355 _ w380]
      tunnel: [FALSE FALSE FALSE TRUE] -> w327
      tunnel: [Data_Producer_States."Read Data" Data_Producer_States."Default" T16."Default" Data_Producer_States."Default"] -> w321
      frame "Read Data" {
        # "Send Raw Data to the Consumer Loop"
        # "Reading Data Check"
        # "Sample Rate"
        n116 = call "Functional Global I32.vi"("Enum"=enum16{"Set Data", "Get Data"}."Get Data") -> ("Integer"=w339:i32)  [unwired: 10 in]
        n117 = Divide(x=w339, y=10) -> (x/y=w338:dbl)
        n118 = call-poly <vilib>:"DAQmxBase Read.vi"("task/channels in"=w352, "number of samples per channel"=w338, "timeout"=100.0, "error in"=w351) -> ("task out"=w350:refnum<k21>, "data"=w337:dbl[][], "error out"=w349:errorcluster)  [unwired: 9 in]
        n119 = Enqueue Element(queue=w348, element=w337, error in (no error)=w347) -> (queue out=w346:refnum<queue>, error out=w345:errorcluster)  [unwired: 1 in, 1 out]
      }
      frame "Default", Default {
      }
      frame "Set Sample Clock" {
        w360 = 10123 items=["Finite Samples"=10178, "Continuous Samples"=10123, "Hardware Timed Single Point"=12522] ("sample mode")
        n120 = property on="Sample Rate" class="DigNum (strict)"("DisabledEnum"=T7."Disabled and Grayed Out" ("Disabled")) -> ()  [unwired: 2 in, 2 out]
        n121 = call <vilib>:"DAQmxBase Create Task.vi"() -> ("task out"=w374:refnum<k21>, "error out"=w373:errorcluster)  [unwired: 14 in]
        n122 = call-poly <vilib>:"DAQmxBase Create Virtual Channel.vi"("task in"=w374, "physical channels"=tag "Dev1/ai0,Dev1/ai1,Dev1/ai2,Dev1/ai3", "error in"=w373) -> ("task out"=w371:refnum<k21>, "error out"=w372:errorcluster)  [unwired: 11 in]
        n123 = call-poly <vilib>:"DAQmxBase Timing.vi"("task/channels in"=w371, "sample mode"=w360, "rate"="Sample Rate", "error in"=w372) -> ("task out"=w370:refnum<k21>, "error out"=w369:errorcluster)  [unwired: 10 in]
        n124 = call <vilib>:"DAQmxBase Start Task.vi"("task/channels in"=w370, "error in"=w369) -> ("task out"=w368:refnum<k21>, "error out"=w359:errorcluster)  [unwired: 12 in]
        n125 = call "Functional Global I32.vi"("Enum"=enum16{"Set Data", "Get Data"}."Set Data", "Integer In"="Sample Rate") -> ()  [unwired: 9 in, 1 out]
        n126 = call <vilib>:"Simple Error Handler.vi"("error in (no error)"=w359) -> ()  [unwired: 4 in, 5 out]
      }
      frame "Exit" {
      }
    }
    n127 = Get Notifier Status(notifier=w318, error in (no error)=w317) -> (current notification=w319:bool)  [unwired: 4 out]
    n128 = Or(x=w327, y=w319) -> (x .or. y?=w320:bool)
  }
  n129 = Release Queue(queue=w31, error in (no error)=w30) -> (error out=w24:errorcluster)  [unwired: 1 in, 2 out]
  n130 = call <vilib>:"DAQmxBase Clear Task.vi"("task in"=w26, "error in"=w25) -> ("error out"=w23:errorcluster)  [unwired: 13 in]
  n131 = Merge Errors(w24, w23) -> (w22:errorcluster)
  n132 = call <vilib>:"Simple Error Handler.vi"("error in (no error)"=w22) -> ()  [unwired: 4 in, 5 out]
